vi "Close File.vi"(8 "error in (no error)":errorcluster, 11 "BLF File":refnum<class "Read Write BLF.lvclass">) -> (0 "error out":errorcluster, 3 "BLF Path":path)   [LabVIEW 2015, in "Read Write BLF.lvclass"]
doc: "This VI will close the BLF file reference, and return the file path that was used.\n\n-------------\nBrian Hoover (Hooovahh)"
uses:
  Read Write BLF.lvclass
  Read Write BLF.lvclass/Read Write BLF.ctl
  <vilib>/Utility/error.llb/Error Cluster From Error Code.vi
  <vilib>/Utility/file.llb/Application Directory.vi
  <vilib>/ErrorRing/Error Ring.xnode
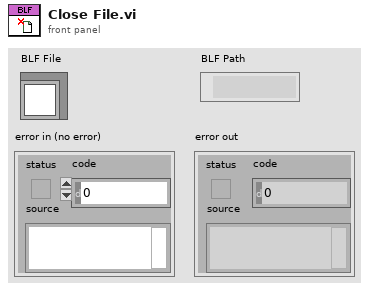
[diagram p1: front panel]
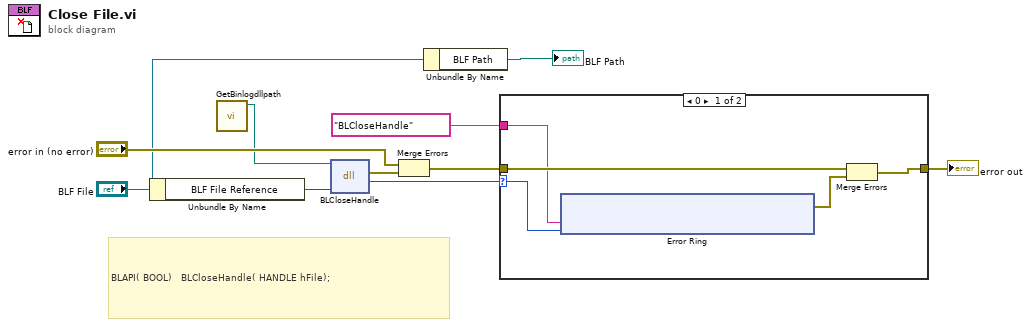
[diagram p0: block diagram]
diagram:
  # "BLAPI( BOOL)   BLCloseHandle( HANDLE hFile);"
  n1 = Unbundle By Name("BLF File") -> ("BLF File Reference"=w4:u32)
  n2 = call "GetBinlogdllpath.vi"() -> ("dup path"=w1:path)  [unwired: 11 in]
  n3 = dll-call lib="PTH2Vabs E自开发软件X-CAN项目 X-CAN离线分析平台 V2.2.8.0BLFbinlog.*" fn="BLCloseHandle"(path in=w1, "hFile"=w4) -> (error out=w10:errorcluster, "返回类型"=w5:i32)  [unwired: 3 in, 1 out]
  n4 = Merge Errors("error in (no error)", w10) -> (w6:errorcluster)
  n5 = Unbundle By Name("BLF File") -> ("BLF Path"=→"BLF Path":path)
  n6 = case shown="0" w5 {
    selector: w5 -> [w13 _]
    tunnel: w6 -> [w15 w24]
    tunnel: [w14 w24] -> w7
    tunnel: "BLCloseHandle" -> [w12 _]
    frame 0 {
      n7 = xnode "Error Ring"("参数 0"=w12, "参数 1"=w13) -> ("错误输出"=w11:errorcluster)
      n8 = Merge Errors(w15, w11) -> (w14:errorcluster)
    }
    frame Default {
    }
  }
  "error out" <- w7
